vi "Write yPointingCorrection_arcsec.vi"(8 "error in (no error)":errorcluster, 10 "yPointingCorrection_arcsec":dbl[unit] min=-0.0048481368110953596 max=0.0048481368110953596, 11 "ADCPointingCorrectionOffsets in":refnum<class "ADCPointingCorrectionOffsets.lvclass">) -> (0 "error out":errorcluster, 3 "ADCPointingCorrectionOffsets out":refnum<class "ADCPointingCorrectionOffsets.lvclass">)   [LabVIEW 2014, in "TCSDataDefinitions.lvlib" / "TCSAtmosphericDispersionCommand.lvlib" / "ADCPointingCorrectionOffsets.lvclass"]
uses:
  ADCPointingCorrectionOffsets.lvclass
  ADCPointingCorrectionOffsets.lvclass/ADCPointingCorrectionOffsets.ctl
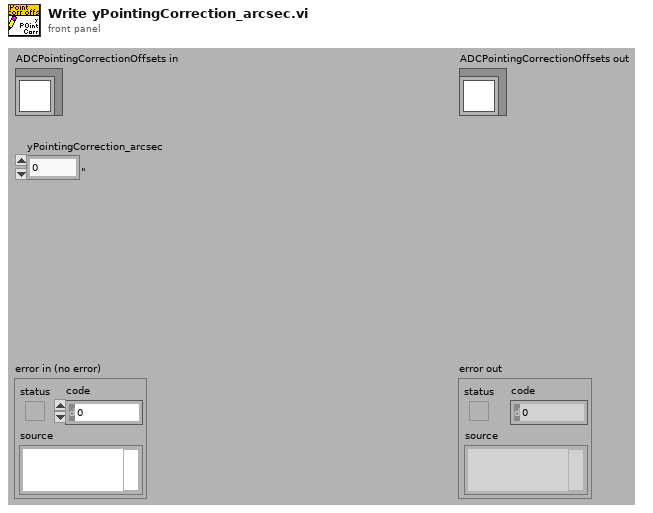
[diagram p1: front panel]
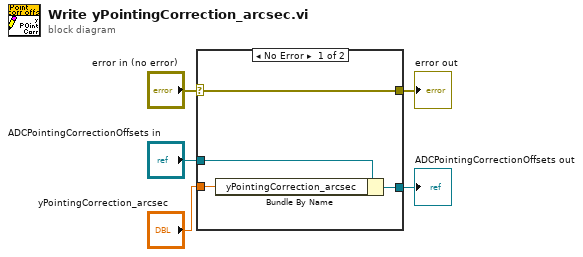
[diagram p0: block diagram]
diagram:
  n1 = case shown="No Error" "error in (no error)" {
    selector: "error in (no error)" -> [w9 w10]
    tunnel: [w9 w10] -> w4
    tunnel: [w7 w11] -> w2
    tunnel: "ADCPointingCorrectionOffsets in" -> [w8 w11]
    tunnel: "yPointingCorrection_arcsec" -> [w6 _]
    frame No Error {
      n2 = Bundle By Name(cluster=w8, "yPointingCorrection_arcsec"=w6) -> (w7:refnum<class "ADCPointingCorrectionOffsets.lvclass">)
    }
    frame Error {
    }
  }
  "error out" <- w4
  "ADCPointingCorrectionOffsets out" <- w2
